vi "SCT Handle Data Type Change.vi"(4 "default types":T2, 6 "feature pack info":T8, 8 "error in (no error)":errorcluster, 9 "OldVal":i32, 10 "state variables in":T4, 11 "Variable Dialog Controls in":T1) -> (0 "error out":errorcluster, 2 "state variables out":T4, 3 "Variable Dialog Controls out":T1)   [LabVIEW 2016]
uses:
  <resource>/dialog/variable/SCT Variable Dialog Controls.ctl
  <resource>/dialog/variable/SCT Feature Pack Info.ctl
  <resource>/dialog/variable/SCT Message User Event.ctl
  <resource>/dialog/variable/SCT Message.ctl
  <vilib>/variable/Type Descriptor.ctl
  <resource>/dialog/variable/SCT Attributes.ctl
  <resource>/dialog/variable/SCT Attributes Event.ctl
  <resource>/dialog/variable/SCT State Variables.ctl
  <resource>/dialog/variable/SCT Feature State.ctl
  <resource>/dialog/variable/SCT Variable Changes.ctl
  <resource>/dialog/variable/SCT Attribute Changes.ctl
  <resource>/dialog/variable/SCT Default Types.ctl
  <vilib>/variable/NI_Variable.lvlib
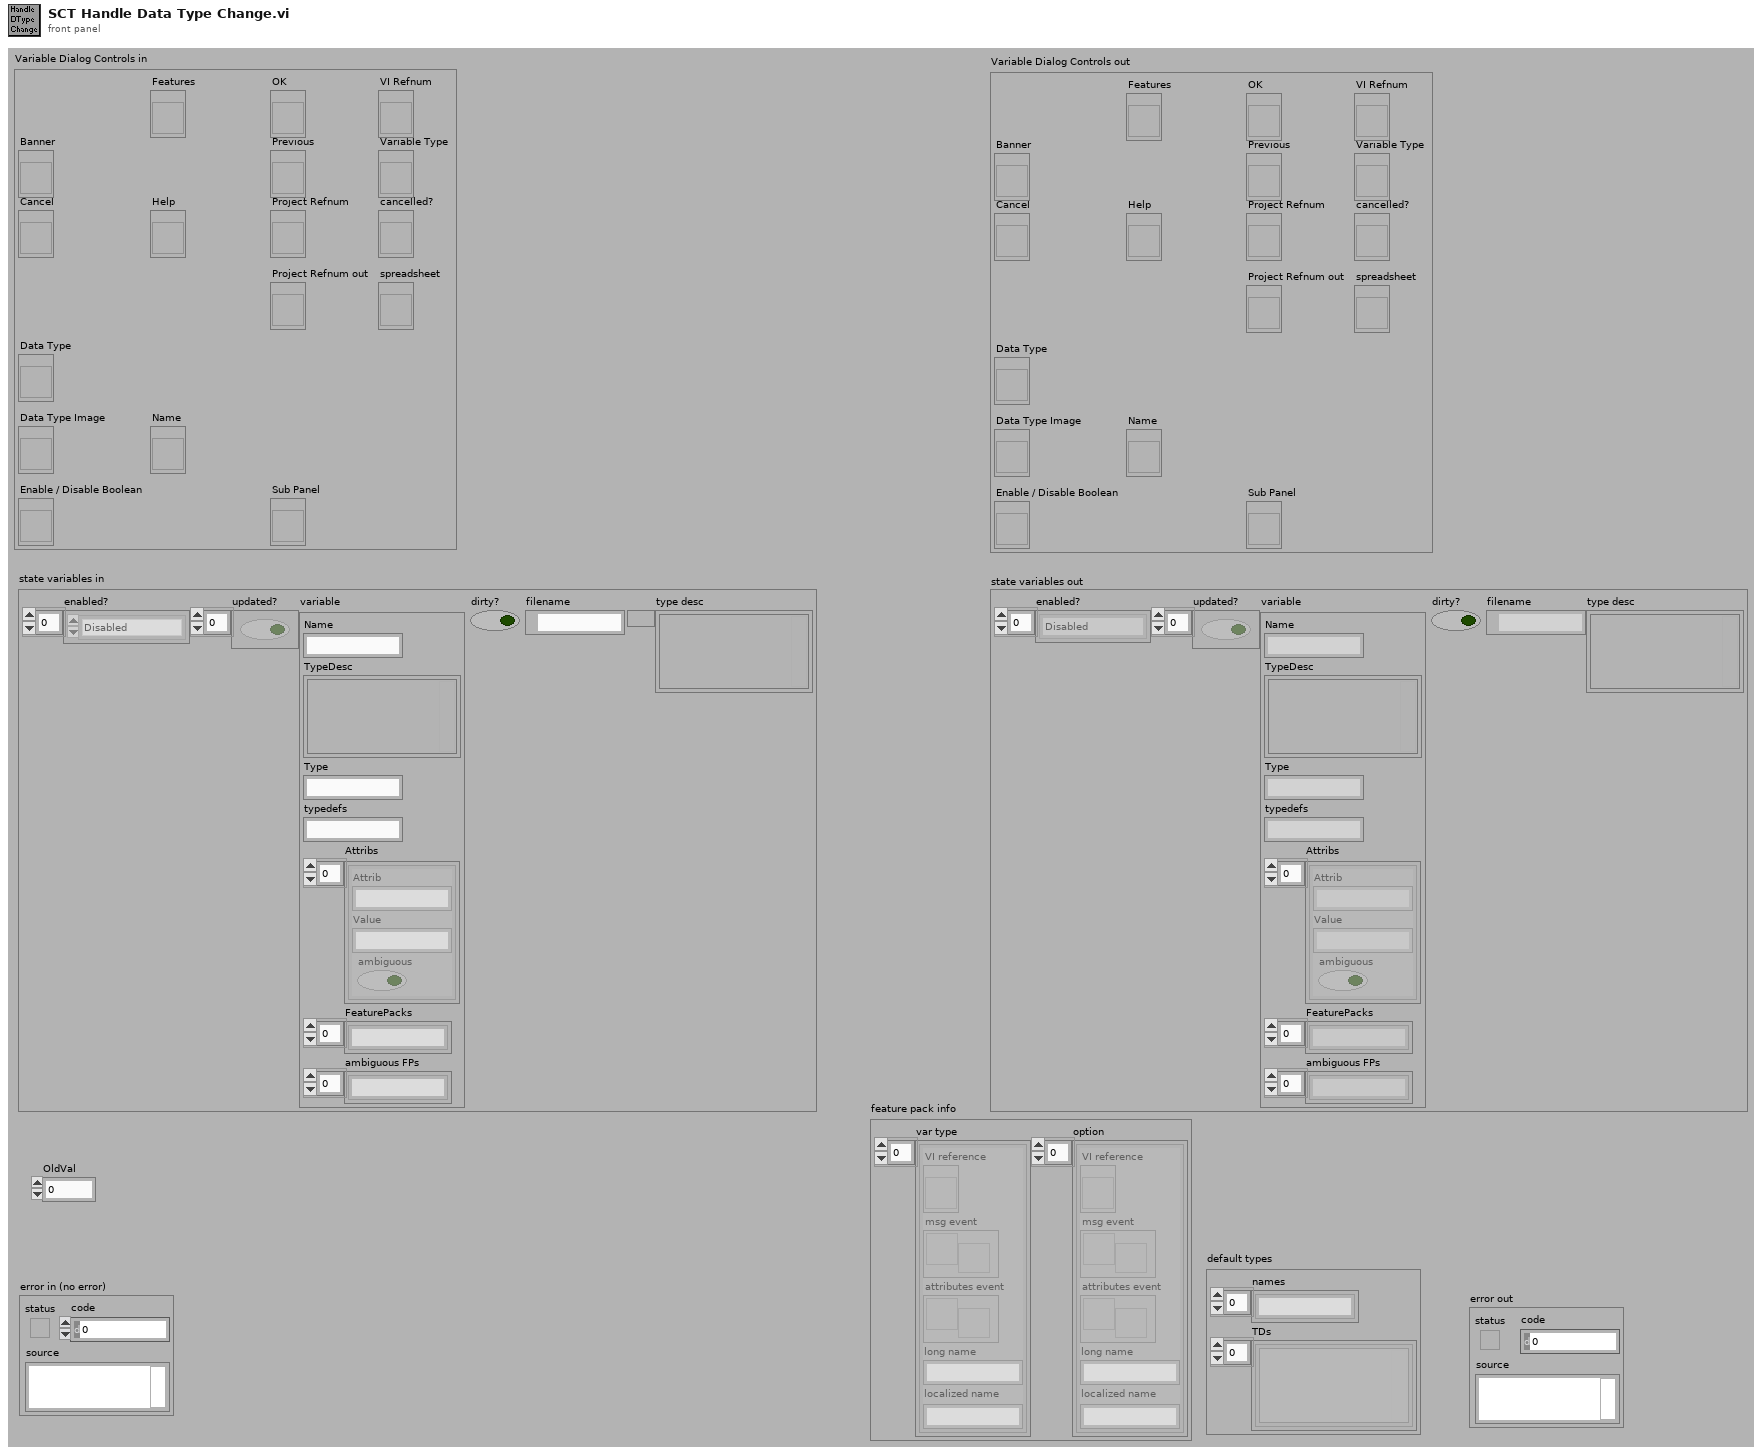
[diagram p1: front panel]
types:
  T1 = typedef "SCT Variable Dialog Controls.ctl" = cluster{"Banner":refnum<vi>, "Cancel":refnum<vi>, "Data Type":refnum<vi>, "Data Type Image":refnum<vi>, "Enable / Disable Boolean":refnum<vi>, "Features":refnum<vi>, "Help":refnum<vi>, "Name":refnum<vi>, "OK":refnum<vi>, "Previous":refnum<vi>, "Project Refnum":refnum<vi>, "Project Refnum out":refnum<vi>, "Sub Panel":refnum<vi>, "VI Refnum":refnum<vi>, "Variable Type":refnum<vi>, "cancelled?":refnum<vi>, "spreadsheet":refnum<vi>}
  T2 = typedef "SCT Default Types.ctl" = cluster{"names":string[], "TDs":T3[]}
  T3 = typedef "NI_Variable.lvlib/Type Descriptor.ctl" = cluster{"Variant":variant}
  T4 = typedef "SCT State Variables.ctl" = cluster{"enabled?":T5[], "updated?":bool[], "variable":T6, "dirty?":bool, "filename":path, "type desc":T3}
  T5 = typedef "SCT Feature State.ctl" = enum16{"Disabled", "Enabled", "Ambiguous", "Grayed", "MultiSelectConst"}
  T6 = typedef "SCT Variable Changes.ctl" = cluster{"Name":string, "TypeDesc":T3, "Type":string, "typedefs":string, "Attribs":T7, "FeaturePacks":string[], "ambiguous FPs":string[]}
  T7 = typedef "SCT Attribute Changes.ctl" = cluster{"Attrib":string, "Value":string, "ambiguous":bool}[]
  T8 = typedef "SCT Feature Pack Info.ctl" = cluster{"var type":cluster{"VI reference":refnum<vi>, "msg event":T9, "attributes event":T10, "long name":string, "localized name":string}[], "option":cluster{"VI reference":refnum<vi>, "msg event":T9, "attributes event":T10, "long name":string, "localized name":string}[]}
  T9 = typedef "SCT Message User Event.ctl" = refnum<user-event>
  T10 = typedef "SCT Attributes Event.ctl" = refnum<user-event>
  T11 = typedef "SCT Message.ctl" = cluster{"request type":enum16{"No Message", "New Data Type", "New Variable", "Request Values", "Shutdown", "Broadcast", "Show Help"}, "name":string, "type descriptor":T3, "scope":string, "attributes":T12, "broadcast value":variant}
  T12 = typedef "SCT Attributes.ctl" = cluster{"name":string, "value":string, "ambiguous?":bool}[]
  T13 = cluster{"VI reference":refnum<vi>, "msg event":T9, "attributes event":T10, "long name":string, "localized name":string}[]
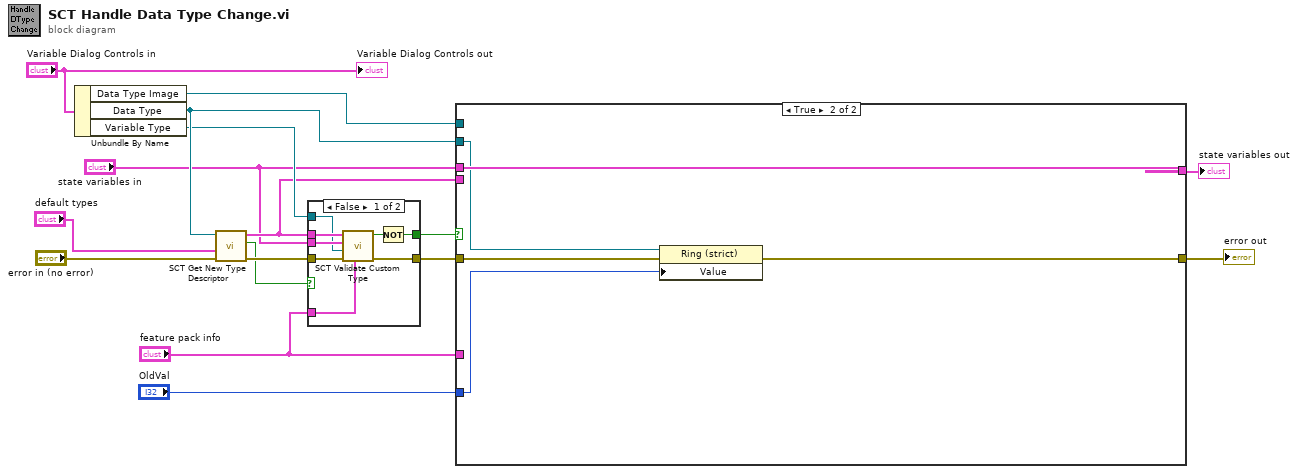
[diagram p0: block diagram]
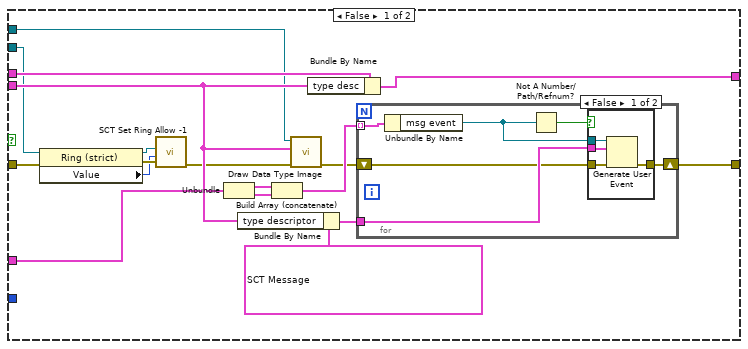
[diagram p3: hidden frame]
diagram:
  n1 = Unbundle By Name("Variable Dialog Controls in") -> ("Data Type Image"=w16:refnum<vi>, "Data Type"=w15:refnum<vi>, "Variable Type"=w14:refnum<vi>)
  n2 = call <resource>:"SCT Get New Type Descriptor.vi"("error in"="error in (no error)", "default types"="default types", "Data Type"=w15) -> ("error out"=w9:errorcluster, "Bounce back"=w6:bool, "new type descriptor"=w11:T3)  [unwired: 6 in]
  n3 = case shown="False" w6 {
    selector: w6 -> [_ w26]
    tunnel: w14 -> [w19 _]
    tunnel: w11 -> [w23 _]
    tunnel: "state variables in" -> [w24 _]
    tunnel: "feature pack info" -> [w20 _]
    tunnel: [w22 w26] -> w7
    tunnel: w9 -> [w18 w25]
    tunnel: [w17 w25] -> w10
    frame False {
      n4 = call <resource>:"SCT Validate Custom Type.vi"("feature pack info"=w20, "error in (no error)"=w18, "Variable Type"=w19, "state variables out"=w24, "new type descriptor"=w23) -> ("error out"=w17:errorcluster, "valid?"=w21:bool)  [unwired: 5 in]
      n5 = Not(x=w21) -> (.not. x?=w22:bool)
    }
    frame True {
    }
  }
  n6 = case shown="True" w7 {
    tunnel: "feature pack info" -> [w35 _]
    tunnel: w11 -> [w37 _]
    tunnel: w15 -> [w30 w56]
    tunnel: "OldVal" -> [_ w57]
    tunnel: "state variables in" -> [w36 w60]
    tunnel: [w38 w60] -> w3
    tunnel: w10 -> [w32 w59]
    tunnel: [w33 w58] -> w12
    tunnel: w16 -> [w27 _]
    frame False {
      n7 = property class="Ring (strict)"(reference=w30, error in=w32) -> (reference out=w29:refnum<vi>, error out=w31:errorcluster, "Value"=w28:i32)
      n8 = call <resource>:"SCT Set Ring Allow -1.vi"("error in (no error)"=w31, "index"=w28, "ring"=w29) -> ("error out"=w34:errorcluster)  [unwired: 7 in, 1 out]
      n9 = Unbundle(w35) -> ("var type"=w44:T13, "option"=w43:T13)
      n10 = Bundle By Name(cluster=T11 {"request type"=enum."New Data Type", "name"="", "type descriptor"={"Variant"=variant}, "scope"="", "attributes"=[], "broadcast value"=variant} ("event data"), "type descriptor"=w37) -> (w41:T11)
      n11 = Build Array (concatenate)(w44, w43) -> (w42:T13)
      n12 = call <vilib>:"Draw Data Type Image.vi"("error in (no error)"=w34, "type descriptor"=w37, "Data Type Image"=w27) -> ("error IO"=w39:errorcluster)  [unwired: 8 in]
      n13 = Bundle By Name(cluster=w36, "type desc"=w37) -> (w38:T4)
      n14 = for {
        tunnel: w42 -> [w50] mode=indexing
        tunnel: w41 -> [w49]
        shift-right: [w45] -> w33
        shift-left: w39 -> [w46]
        n15 = Unbundle By Name(w50) -> ("msg event"=w48:T9)
        n16 = Not A Number/Path/Refnum?(number/path/refnum=w48) -> (NaN/Path/Refnum?=w47:bool)
        n17 = case shown="False" w47 {
          tunnel: w49 -> [w54 _]
          tunnel: w48 -> [w53 _]
          tunnel: w46 -> [w52 w55]
          tunnel: [w51 w55] -> w45
          frame False {
            n18 = Generate User Event(user event=w53, event data cluster=w54, error in=w52) -> (error out=w51:errorcluster)  [unwired: 1 in, 1 out]
          }
          frame True {
          }
        }
      }
    }
    frame True {
      n19 = property class="Ring (strict)"(reference=w56, error in=w59, "Value"=w57) -> (error out=w58:errorcluster)  [unwired: 1 out]
    }
  }
  "error out" <- w12
  "state variables out" <- w3
  "Variable Dialog Controls out" <- "Variable Dialog Controls in"
